vi "GetResult.vi"(8 "error in (no error)":errorcluster, 11 "AbstractBuilder in":refnum<class "AbstractBuilder.lvclass">) -> (0 "error out":errorcluster, 2 "BrowerComponent":refnum<class "BrowerComponent.lvclass">, 3 "AbstractBuilder out":refnum<class "AbstractBuilder.lvclass">)   [LabVIEW 2015, in "AbstractBuilder.lvclass"]
uses:
  AbstractBuilder.lvclass
  BrowerComponent/BrowerComponent/BrowerComponent.lvclass
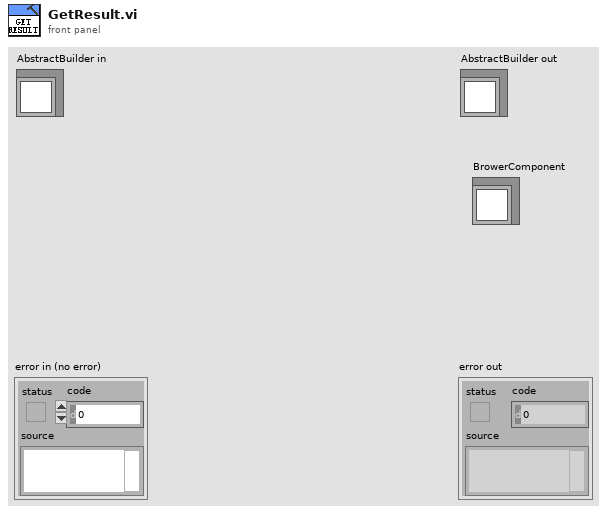
[diagram p1: front panel]
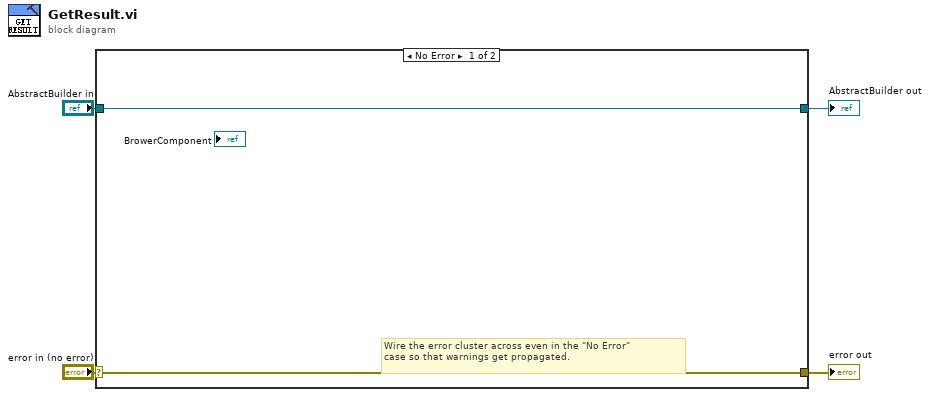
[diagram p0: block diagram]
diagram:
  n1 = case shown="No Error" "error in (no error)" {
    selector: "error in (no error)" -> [w5 w8]
    tunnel: [w5 w8] -> w3
    tunnel: [w6 w7] -> w1
    tunnel: "AbstractBuilder in" -> [w6 w7]
    frame No Error {
      # "Wire the error cluster across even in the \"No Error\"\ncase so that warnings get propagated."
    }
    frame Error {
    }
  }
  "error out" <- w3
  "AbstractBuilder out" <- w1
